vi "Util.Pic.GIF.Block.PackUnpack__ogtk.vi"(6 "Calling routine":string, 8 "error in (no error)":errorcluster, 9 "StartIndex":i32, 10 "BlockBytes in":u8[](array[numeric]), 11 "Pack/Unpack (T/F)":bool) -> (0 "error out":errorcluster, 1 "LastIndex":i32, 2 "BlockBytes out":u8[](array[numeric]) format="%.0x")   [LabVIEW 2020]
panel:
  # "GIF.Block.PackUnpack.vi\n\nPacks or Unpacks a data-stream composed of GIF \"Blocks.\nA Block is a sequence of bytes beginning with a length-byte followed by data bytes.\nThe length-byte can be from 0 to 255 and specifies the number of bytes that follow. (The length-byte is not included in length.)\n\"Pack\"ing produces a data stream that includes length-bytes.\n\"Unpack\"ing removes length-bytes from the data-stream.\n\nPlease visit http://www.OpenG.org to learn about the\nOpen Source LabVIEW software movement.\n\nNOTICE -- YOU MUST LEAVE THIS NOTICE IN PLACE.  PER THE TERMS OF THE LICENSE BELOW, YOU MAY SUBLICENSE THIS SOFTWARE \nIN ANY WAY THAT DOES NOT CONFLICT WITH THIS LICENSE.\n\n### BSD License (http://www.opensource.org/licenses/bsd-license.php) Begin ###\n \nCopyright (c) 2007, Bill Clench <bclench@yahoo.com>\n\nAll rights reserved.\n\nRedistribution and use in source and binary forms, with or without modification, are permitted provided that the following conditions are met:\n\n    * Redistributions of source code must retain the above copyright notice, this list of conditions and the following disclaimer.\n    * Redistributions in binary form must reproduce the above copyright notice, this list of conditions and the following disclaimer in the \n       documentation and/or other materials provided with the distribution.\n    * Neither the name of SciWare, James Kring, Inc., nor the names of its contributors may be used to endorse or promote products derived \n       from this software without specific prior written permission.\n\nTHIS SOFTWARE IS PROVIDED BY THE COPYRIGHT HOLDERS AND CONTRIBUTORS \"AS IS\" AND ANY EXPRESS OR IMPLIED WARRANTIES, \nINCLUDING, BUT NOT LIMITED TO, THE IMPLIED WARRANTIES OF MERCHANTABILITY AND FITNESS FOR A PARTICULAR PURPOSE ARE \nDISCLAIMED. IN NO EVENT SHALL THE COPYRIGHT OWNER OR CONTRIBUTORS BE LIABLE FOR ANY DIRECT, INDIRECT, INCIDENTAL,\n SPECIAL, EXEMPLARY, OR CONSEQUENTIAL DAMAGES (INCLUDING, BUT NOT LIMITED TO, PROCUREMENT OF SUBSTITUTE GOODS OR \nSERVICES; LOSS OF USE, DATA, OR PROFITS; OR BUSINESS INTERRUPTION) HOWEVER CAUSED AND ON ANY THEORY OF LIABILITY, \nWHETHER IN CONTRACT, STRICT LIABILITY, OR TORT (INCLUDING NEGLIGENCE OR OTHERWISE) ARISING IN ANY WAY OUT OF THE USE \nOF THIS SOFTWARE, EVEN IF ADVISED OF THE POSSIBILITY OF SUCH DAMAGE.\n\n### BSD License End ###"
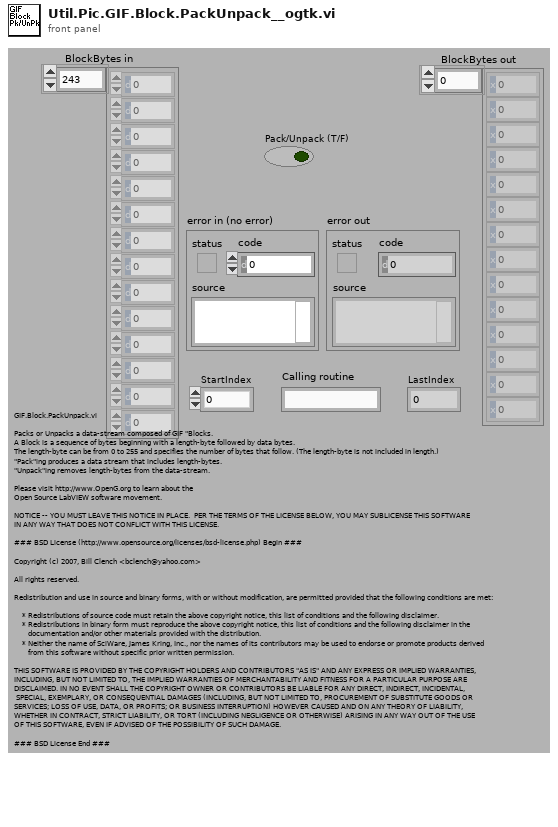
[diagram p1: front panel]
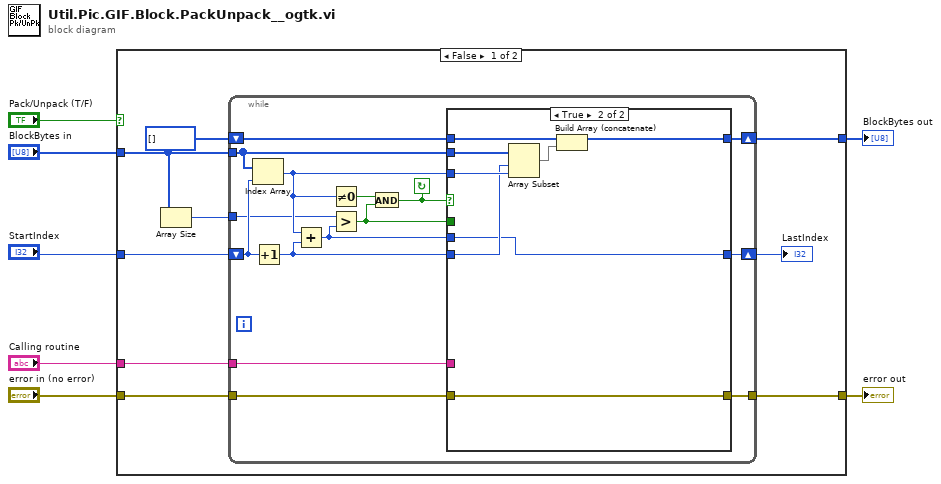
[diagram p0: block diagram]
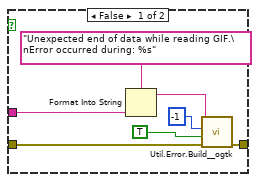
[diagram p3: hidden frame]
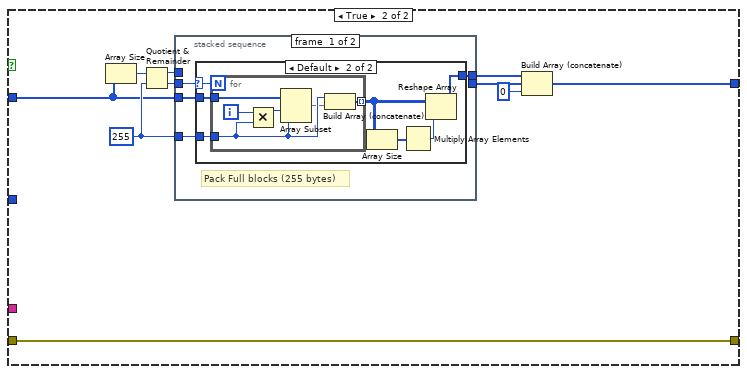
[diagram p4: hidden frame]
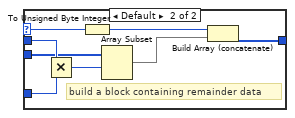
[diagram p7: hidden frame]
diagram:
  n1 = case shown="False" "Pack/Unpack (T/F)" {
    tunnel: "BlockBytes in" -> [w11 w55]
    tunnel: [w14 w56] -> w7
    tunnel: "StartIndex" -> [w13 _]
    tunnel: "error in (no error)" -> [w10 w54]
    tunnel: "Calling routine" -> [w9 _]
    tunnel: [w8 w54] -> w1
    frame False {
      n2 = Array Size(array=w11) -> (size(s)=w12:i32)
      n3 = while {
        shift-right: [w29] -> w15
        shift-left: w13 -> [w27]
        tunnel: w11 -> [w31]
        shift-right: [w28] -> w14
        shift-left: u8[] [] -> [w30]
        tunnel: w12 -> [w23]
        tunnel: w10 -> [w21]
        tunnel: w9 -> [w19]
        tunnel: [w18] -> w8
        stop <- w17 continue-if-true
        n4 = Index Array(array=w31, index=w27) -> (element=w25:u8)
        n5 = Increment(x=w27) -> (x+1=w26:i32)
        n6 = Add(x=w25, y=w26) -> (x+y=w24:i32)
        n7 = Not Equal To 0?(x=w25) -> (x != 0?=w22:bool)
        n8 = Greater?(x=w23, y=w24) -> (0:w20:bool)
        n9 = And(x=w22, y=w20) -> (x .and. y?=w17:bool)
        n10 = case shown="True" w17 {
          tunnel: w31 -> [_ w53]
          tunnel: w30 -> [w37 w52]
          tunnel: w25 -> [_ w50]
          tunnel: [w36 w47] -> w29
          tunnel: [w37 w49] -> w28
          tunnel: w26 -> [w36 w48]
          tunnel: w24 -> [_ w47]
          tunnel: w21 -> [w33 w46]
          tunnel: w20 -> [w35 _]
          tunnel: w19 -> [w34 _]
          tunnel: [w32 w46] -> w18
          frame False {
            # "Return next index\nSkip 0 (terminate) byte"
            n11 = case shown="True" w35 {
              tunnel: w34 -> [w43 _]
              tunnel: w33 -> [w42 w45]
              tunnel: [w41 w45] -> w32
              frame False {
                n12 = Format Into String(format string="Unexpected end of data while reading GIF.\nError occurred during: %s", w43) -> (resulting string=w40:string)  [unwired: 2 in, 1 out]
                n13 = call <userlib>:"Util.Error.Build__ogtk.vi"("error in (no error)"=w42, "Status"=TRUE, "code"=-1, "Source"=w40) -> ("error out"=w41:errorcluster)  [unwired: 7 in]
              }
              frame True {
              }
            }
          }
          frame True {
            n14 = Array Subset(array=w53, index=w48, length=w50) -> (w51:u8[])
            n15 = Build Array (concatenate)(w52, w51) -> (w49:u8[])
          }
        }
      }
      "LastIndex" <- w15
    }
    frame True {
      w60 = u8 255
      n16 = Array Size(array=w55) -> (size(s)=w58:i32)
      n17 = Quotient & Remainder(x=w58, y=w60) -> (x-y*floor(x/y)=w62:i32, floor(x/y)=w59:i32)
      n18 = stacked-sequence {
        tunnel: w59 -> [w64 w83]
        tunnel: w55 -> [w66 w81]
        tunnel: w60 -> [w67 w82]
        tunnel: [w65 _] -> w61
        tunnel: w62 -> [_ w85]
        tunnel: [_ w84] -> w63
        frame #0 {
          # "Pack Full blocks (255 bytes)"
          n19 = case shown="Default" w64 {
            selector: w64 -> [_ w69]
            tunnel: w67 -> [_ w74]
            tunnel: w66 -> [_ w73]
            tunnel: [_ w68] -> w65
            frame 0 {
            }
            frame Default {
              n20 = for {
                N: w69 -> [_]
                tunnel: w74 -> [w77]
                tunnel: w73 -> [w79]
                tunnel: [w75] -> w72 mode=indexing
                i -> [w80]
                n21 = Multiply(x=w80, y=w77) -> (x*y=w78:i32)
                n22 = Array Subset(array=w79, index=w78, length=w77) -> (w76:u8[])
                n23 = Build Array (concatenate)(w77, w76) -> (w75:u8[])
              }
              n24 = Array Size(array=w72) -> (size(s)=w71:i32[])
              n25 = Multiply Array Elements(1:w71) -> (0:w70:i32)
              n26 = Reshape Array(w72, w70) -> (w68:u8[])
            }
          }
        }
        frame #1 {
          # "pack remaining bytes/block in image"
          n27 = case shown="0" w85 {
            selector: w85 -> [_ w93]
            tunnel: [_ w92] -> w84
            tunnel: w83 -> [_ w91]
            tunnel: w82 -> [_ w90]
            tunnel: w81 -> [_ w88]
            frame 0 {
            }
            frame Default {
              # "build a block containing remainder data"
              n28 = Multiply(x=w91, y=w90) -> (x*y=w87:i32)
              n29 = To Unsigned Byte Integer(number=w93) -> (unsigned 8bit integer=w89:u8)
              n30 = Array Subset(array=w88, index=w87) -> (w86:u8[])  [unwired: 1 in]
              n31 = Build Array (concatenate)(w89, w86) -> (w92:u8[])
            }
          }
        }
      }
      n32 = Build Array (concatenate)(w61, w63, u8 0) -> (w56:u8[])
    }
  }
  "BlockBytes out" <- w7
  "error out" <- w1
